vi "grSim Command.vi"(9 "Robots":T1[](array[typedef]), 10 "isteamyellow":bool=TRUE, 11 "timestamp":dbl format="%#_13g") -> (1 "Array":u8[](array[numeric]))   [LabVIEW 2016]
uses:
  grSim Robot Command.ctl
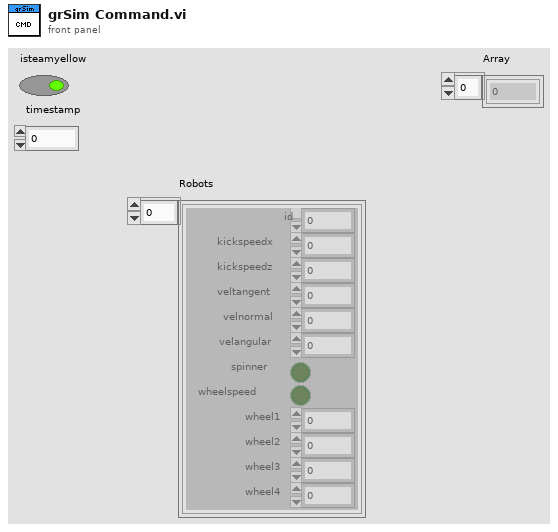
[diagram p1: front panel]
types:
  T1 = typedef "grSim Robot Command.ctl" = cluster{"id":u32, "kickspeedx":sgl, "kickspeedz":sgl, "veltangent":sgl, "velnormal":sgl, "velangular":sgl, "spinner":bool, "wheelspeed":bool, "wheel1":sgl, "wheel2":sgl, "wheel3":sgl, "wheel4":sgl}
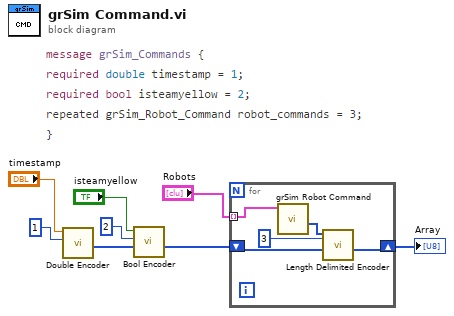
[diagram p0: block diagram]
diagram:
  n1 = call "Double Encoder.vi"("Key"=u32 1, "Value"="timestamp") -> ("Array"=w7:u8[])  [unwired: 9 in]
  n2 = call "Bool Encoder.vi"("Array In"=w7, "Key"=u32 2, "Value"="isteamyellow") -> ("Array"=w3:u8[])  [unwired: 8 in]
  n3 = for {
    shift-right: [w10] -> w2
    shift-left: w3 -> [w11]
    tunnel: "Robots" -> [w13] mode=indexing
    n4 = call "grSim Robot Command.vi"("Robots"=w13) -> ("Array"=w12:u8[])  [unwired: 10 in]
    n5 = call "Length Delimited Encoder.vi"("Array In"=w11, "Key"=u32 3, "Array In 2"=w12) -> ("Array"=w10:u8[])  [unwired: 8 in]
  }
  "Array" <- w2
